vi "ScriptWireTunnels.vi"(9 "i/o terminals":refnum<vi>[](array[refnum]), 10 "CaseStructure in":refnum<vi>, 11 "ControlTerminal in":refnum<vi>) -> (0 "error out":errorcluster)   [LabVIEW 2014]
uses:
  <vilib>/Utility/miscctls.llb/LVBoundsTypeDef.ctl
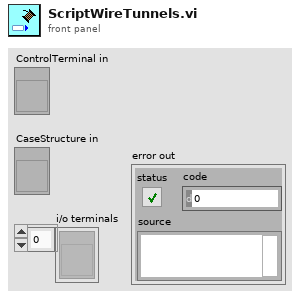
[diagram p1: front panel]
types:
  T1 = typedef "LVBoundsTypeDef.ctl" = cluster{"Width":u32, "Height":u32}
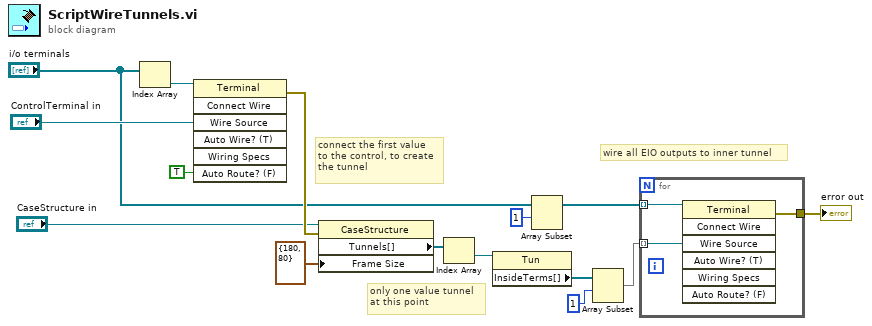
[diagram p0: block diagram]
diagram:
  # "connect the first value\nto the control, to create\nthe tunnel"
  # "wire all EIO outputs to inner tunnel"
  # "only one value tunnel\nat this point"
  n1 = Index Array(array="i/o terminals") -> (element=w11:refnum<vi>)  [unwired: 1 in]
  n2 = invoke on="Invoke Node" class="Terminal" method="Connect Wire"(reference=w11, "Wire Source"="ControlTerminal in", "Auto Route? (F)"=TRUE) -> (error out=w15:errorcluster)  [unwired: 4 in, 6 out]
  n3 = property class="CaseStructure"(reference="CaseStructure in", error in=w15, "Frame Size"=T1 {"Width"=180, "Height"=80}) -> ("Tunnels[]"=w8:refnum<vi>[])  [unwired: 2 out]
  n4 = Index Array(array=w8) -> (element=w10:refnum<vi>)  [unwired: 1 in]
  n5 = property class="Tun"(reference=w10) -> ("InsideTerms[]"=w2:refnum<vi>[])  [unwired: 1 in, 2 out]
  n6 = Array Subset(array="i/o terminals", index=1) -> (w6:refnum<vi>[])  [unwired: 1 in]
  n7 = Array Subset(array=w2, index=1) -> (w1:refnum<vi>[])  [unwired: 1 in]
  n8 = for {
    tunnel: w1 -> [w18] mode=indexing
    tunnel: w6 -> [w17] mode=indexing
    tunnel: [w16] -> w12
    n9 = invoke on="Invoke Node" class="Terminal" method="Connect Wire"(reference=w17, "Wire Source"=w18) -> (error out=w16:errorcluster)  [unwired: 5 in, 6 out]
  }
  "error out" <- w12
